vi "串口INI.vi"(1 "串口参数":T1={"VISA串口名称"="", "波特率"=9600, "停止位"=10, "流控制"=0, "数据位"=8, "奇偶校验"=enum."None", "超时"=2000, "启用终止符？"=FALSE, "终止符"=10} {"终止符" format="%.0x"; "数据位" min=5 max=8 step=1; "流控制" items=["无", "XON/XOFF", "RTS/CTS", "XON/XOFF & RTS/CTS", "DTR/DSR", "XON/XOFF & DTR/DSR"]; "停止位" items=["1.0"=10, "1.5"=15, "2.0"=20]; "波特率" items=["9600"=9600, "115200"=15]}) -> (14 "串口":refnum<visa-resource-name>, 16 "可用？":bool)   [LabVIEW 2019, in "MainPage.lvlib" / "MainPage.lvclass"]
uses:
  MainPage.lvclass
  <vilib>/Instr/_visa.llb/VISA Configure Serial Port (Instr).vi
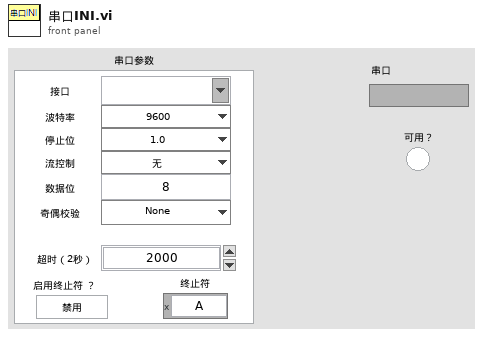
[diagram p1: front panel]
types:
  T1 = cluster{"VISA串口名称":refnum<visa-resource-name>, "波特率":u32, "停止位":u16, "流控制":u16, "数据位":u16, "奇偶校验":enum16{"None", "Odd", "Even", "Mark", "Space"}, "超时":u32, "启用终止符？":bool, "终止符":u8}
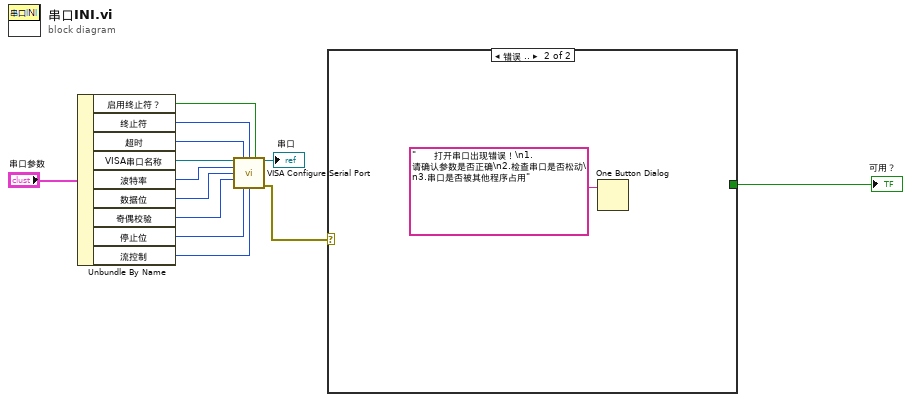
[diagram p0: block diagram]
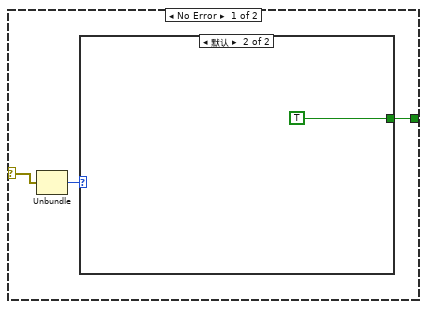
[diagram p2: hidden frame]
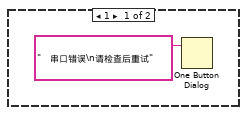
[diagram p3: hidden frame]
diagram:
  n1 = Unbundle By Name("串口参数") -> ("启用终止符？"=w12:bool, "终止符"=w11:u8, "超时"=w10:u32, "VISA串口名称"=w9:refnum<visa-resource-name>, "波特率"=w8:u32, "数据位"=w7:u16, "奇偶校验"=w6:enum16{"None", "Odd", "Even", "Mark", "Space"}, "停止位"=w5:u16, "流控制"=w4:u16)
  n2 = call-poly "VISA Configure Serial Port"("VISA resource name"=w9, "timeout (10sec)"=w10, "termination char\n(0xA = '\\n' = LF)"=w11, "Enable Termination\nChar (T)"=w12, "baud rate (9600)"=w8, "data bits (8)"=w7, "parity (0:none)"=w6, "stop bits (10: 1 bit)"=w5, "flow control (0:none)"=w4) -> ("VISA resource name out"=→"串口":refnum<visa-resource-name>, "error out"=w3:errorcluster)  [unwired: 5 in]
  n3 = case shown="错误 .." w3 {
    selector: w3 -> [w16 _]
    tunnel: [w14 _] -> w2
    frame No Error {
      n4 = Unbundle(w16) -> ("code"=w15:i32)  [unwired: 2 out]
      n5 = case shown="默认" w15 {
        tunnel: [_ TRUE] -> w14
        frame 1 {
          n6 = One Button Dialog(message="   串口错误\n请检查后重试" ("消息")) -> ()  [unwired: 1 in, 1 out]
        }
        frame Default {
        }
      }
    }
    frame Error {
      n7 = One Button Dialog(message="      打开串口出现错误！\n1.请确认参数是否正确\n2.检查串口是否松动\n3.串口是否被其他程序占用" ("消息")) -> ()  [unwired: 1 in, 1 out]
    }
  }
  "可用？" <- w2
